vi "DSF.Shared.Configuration.Channels Configuration.Validate.vi"(8 "error in (no error)":errorcluster, 11 "Channels Configuration in":T1[](array[typedef]) {"offset" format="%d bytes"}) -> (0 "error out":errorcluster, 3 "Channels Configuration out":T1[](array[typedef]) {"offset" format="%d bytes"})   [LabVIEW 2016, in "DSF.Shared.lvlib"]
uses:
  DSF.Shared.lvlib
  Typedefs/DSF.Shared.Typedefs.Configuration.Transfer.Channel Properties.ctl
  Typedefs/DSF.Shared.Typedefs.Data Type.ctl
panel:
  out "invalid index":i32
  out "valid?":bool
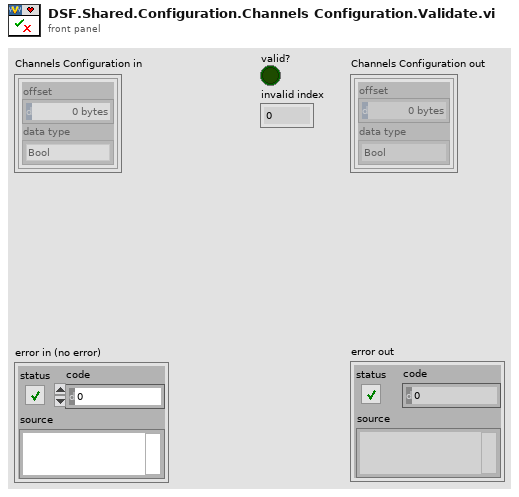
[diagram p1: front panel]
types:
  T1 = typedef "DSF.Shared.lvlib/DSF.Shared.Typedefs.Configuration.Transfer.Channel Properties.ctl" = cluster{"offset":u64, "data type":T2}
  T2 = typedef "DSF.Shared.lvlib/DSF.Shared.Typedefs.Data Type.ctl" = enum8{"Bool", "SGL", "DBL", "I8", "I16", "I32", "I64", "U8", "U16", "U32", "U64"}
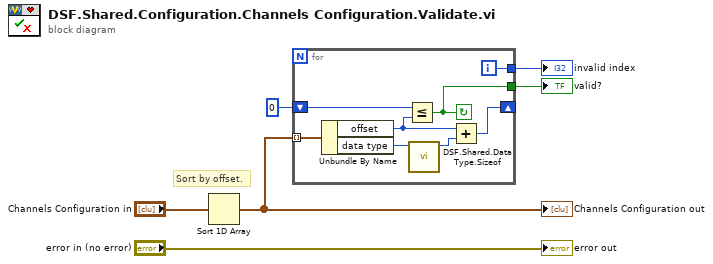
[diagram p0: block diagram]
diagram:
  # "Sort by offset."
  n1 = Sort 1D Array(array="Channels Configuration in") -> (sorted array=w4:T1[])
  "Channels Configuration out" <- w4
  n2 = for {
    tunnel: w4 -> [w14] mode=indexing
    shift-right: [w9] -> _
    shift-left: u64 0 ("offset") -> [w13]
    tunnel: [w8] -> w1
    tunnel: [w7] -> w2
    i -> [w8]
    stop <- w7 continue-if-true
    n3 = Unbundle By Name(w14) -> ("offset"=w11:u64, "data type"=w12:T2)
    n4 = Less Or Equal?(x=w13, y=w11) -> (x <= y?=w7:bool)
    n5 = call "DSF.Shared.Data Type.Sizeof.vi"("data type"=w12) -> ("size in bytes"=w10:u64)  [unwired: 9 in, 1 out]
    n6 = Add(x=w11, y=w10) -> (x+y=w9:u64)
  }
  "valid?" <- w2
  "invalid index" <- w1
  "error out" <- "error in (no error)"
